vi "CAN Stop Schedule.vi"(8 "error in (no error)":errorcluster, 10 "CANIndex":u8, 11 "DevHandle":i32) -> (0 "error out":errorcluster, 3 "function return":i32)   [LabVIEW 2010, in "usb2an.lvlib"]
doc: "int WINAPI CAN_StopSchedule(int DevHandle, unsigned char CANIndex);"
uses:
  usb2an.lvlib
  USB2XXX.dll
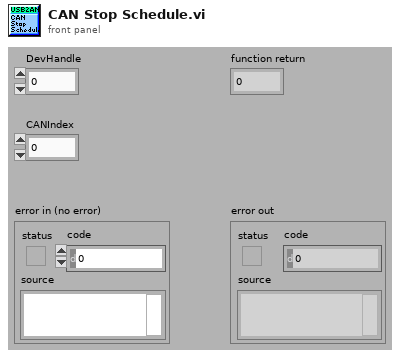
[diagram p1: front panel]
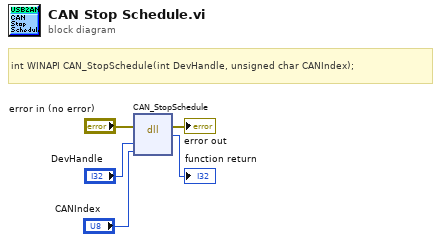
[diagram p0: block diagram]
diagram:
  # "int WINAPI CAN_StopSchedule(int DevHandle, unsigned char CANIndex);"
  n1 = dll-call lib="E:/OtherWork/STM32/USB2XXX_Example/sdk/api/Labview/USB2XXX.*" fn="CAN_StopSchedule"(error in="error in (no error)", "DevHandle"="DevHandle", "CANIndex"="CANIndex") -> (error out=→"error out":errorcluster, →"function return":i32)  [unwired: 4 in, 1 out]
